vi "REPORT_GEAR_prepare_header_for_pdf.vi"(11 "REPORT_GEAR_all_info":T1) -> (3 "report_header":string[][](array[string]))   [LabVIEW 2019]
uses:
  typedef/REPORT_GEAR_all_info.ctl
  typedef/REPORT_GEAR_header_data_display.ctl
  typedef/REPORT_GEAR_statuses.ctl
  _misc/AULocalize/SubVIs/Get Localized Phrase Compact Interface 1D.vi
panel:
  # "GEAR INFO SUMMARY"
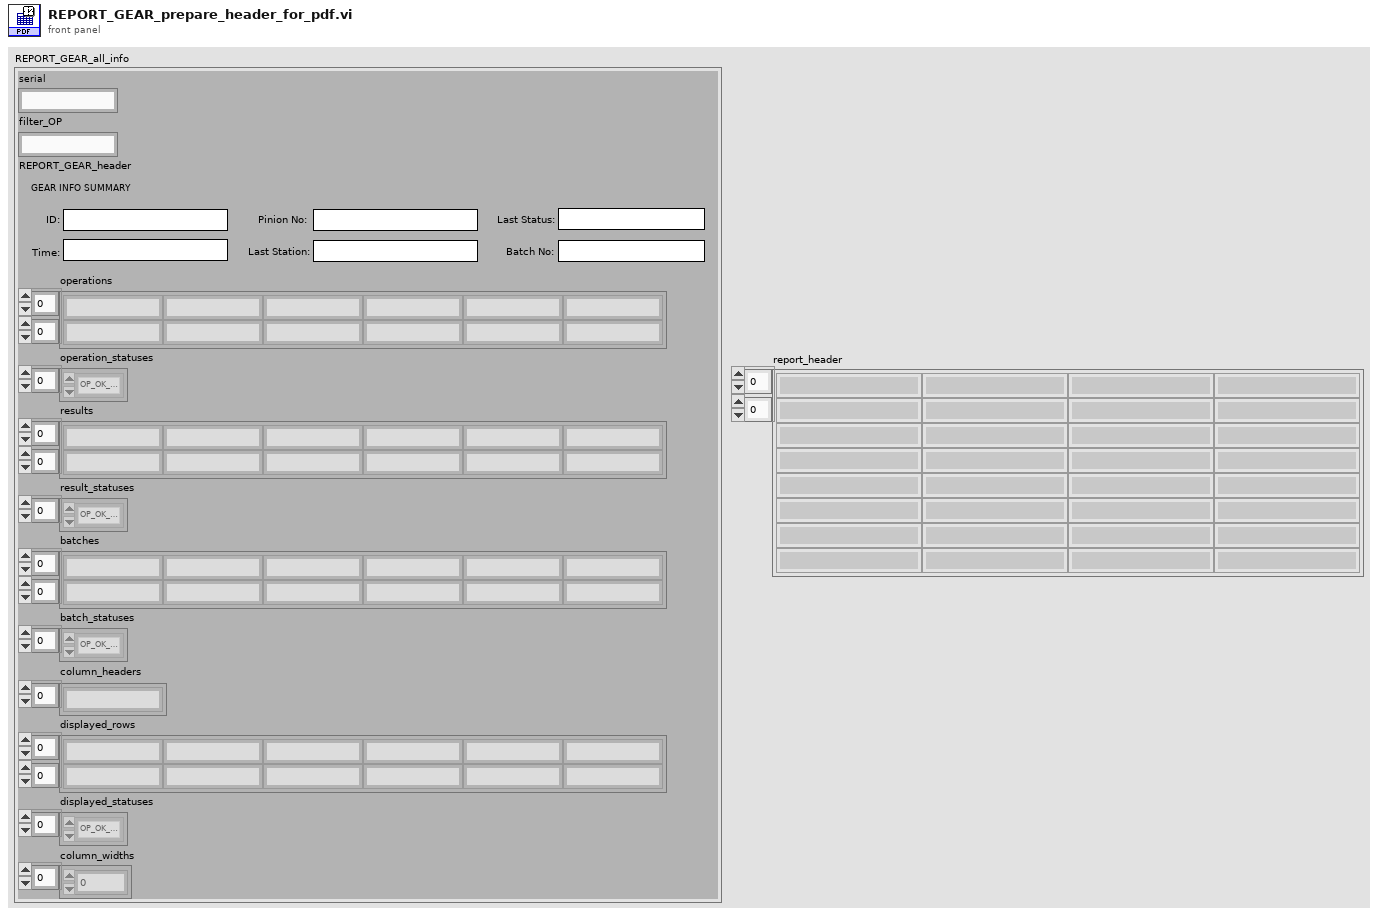
[diagram p1: front panel]
types:
  T1 = typedef "REPORT_GEAR_all_info.ctl" = cluster{"serial":string, "filter_OP":string, "REPORT_GEAR_header":T2, "operations":string[][], "operation_statuses":T3[], "results":string[][], "result_statuses":T3[], "batches":string[][], "batch_statuses":T3[], "column_headers":string[], "displayed_rows":string[][], "displayed_statuses":T3[], "column_widths":i16[]}
  T2 = typedef "REPORT_GEAR_header_data_display.ctl" = cluster{"ID":string, "creation_time":string, "last_station":string, "last_status":string, "pinion_serial":string, "batch_code":string}
  T3 = typedef "REPORT_GEAR_statuses.ctl" = enum16{"OP_OK_hide", "OP_OK_show", "OP_NOK_hide", "OP_NOK_show", "OP_interrupted_hide", "OP_interrupted_show", "OP_in_operation_hide", "OP_in_operation_show", "OP_unexpected_hide", "OP_unexpected_show", "RE_REAL_OK", "RE_REAL_NOK", "RE_STRING", "RE_sub_header", "RE_no_data", "RE_unexpected", "BA_sub_header", "BA_data", "BA_no_data"}
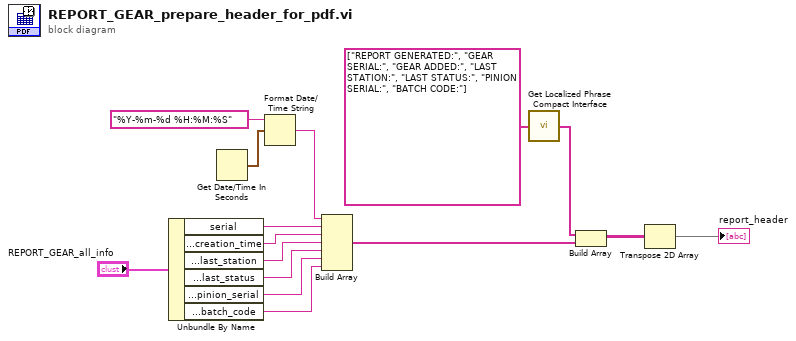
[diagram p0: block diagram]
diagram:
  n1 = Unbundle By Name("REPORT_GEAR_all_info") -> ("serial"=w9:string, "REPORT_GEAR_header.creation_time"=w7:string, "REPORT_GEAR_header.last_station"=w8:string, "REPORT_GEAR_header.last_status"=w6:string, "REPORT_GEAR_header.pinion_serial"=w5:string, "REPORT_GEAR_header.batch_code"=w4:string)
  n2 = Get Date/Time In Seconds() -> (seconds since 1Jan1904=w14:timestamp)
  n3 = Format Date/Time String(time format string (%c)="%Y-%m-%d %H:%M:%S", seconds (now)=w14) -> (date/time string=w2:string)  [unwired: 1 in]
  n4 = Build Array(w2, w9, w7, w8, w6, w5, w4) -> (w3:string[])
  n5 = call-poly "Get Localized Phrase Compact Interface.vi"("Key"=string[] ["REPORT GENERATED:", "GEAR SERIAL:", "GEAR ADDED:", "LAST STATION:", "LAST STATUS:", "PINION SERIAL:", "BATCH CODE:"]) -> ("Translated Phrase"=w1:string[])
  n6 = Build Array(w1, w3) -> (w12:string[][])
  n7 = Transpose 2D Array(2D array=w12) -> (transposed array=→"report_header":string[][])
